vi "WindSensor.vi"   [LabVIEW 2018]
uses:
  WindSensorSignatureSettings.ctl
types:
  T1 = typedef "WindSensorSignatureSettings.ctl" = cluster{"DataFIFO":refnum<k21>, "CalculateFIFO":refnum<k21>, "SignatureFIFO":refnum<k21>}
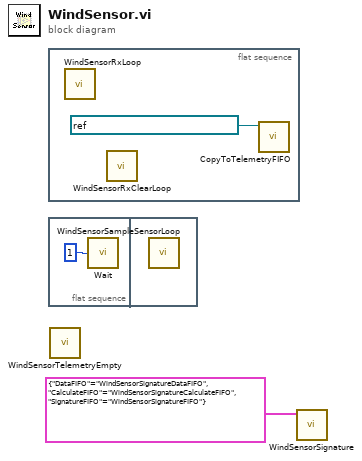
[diagram p0: block diagram]
diagram:
  n1 = flat-sequence {
    frame #0 {
      n2 = call "WindSensorRxLoop.vi"() -> ()  [unwired: 12 in]
      n3 = call "WindSensorRxClearLoop.vi"() -> ()  [unwired: 12 in]
      n4 = call "CopyToTelemetryFIFO.vi"("SourceFIFO"=refnum<k21> "WindSensorTelemetryFIFO") -> ()  [unwired: 11 in]
    }
  }
  n5 = flat-sequence {
    frame #0 {
      n6 = call "Wait"("Count(mSec)"=u8 1) -> ()  [unwired: 1 out]
    }
    frame #1 {
      n7 = call "WindSensorSampleSensorLoop.vi"() -> ()  [unwired: 12 in]
    }
  }
  n8 = call "WindSensorTelemetryEmpty.vi"() -> ()  [unwired: 12 in]
  n9 = call "WindSensorSignature.vi"("WindSensorSignatureSettings"=T1 {"DataFIFO"="WindSensorSignatureDataFIFO", "CalculateFIFO"="WindSensorSignatureCalculateFIFO", "SignatureFIFO"="WindSensorSignatureFIFO"}) -> ()  [unwired: 11 in]
